vi "IMAQ-test.vi"() -> ()   [LabVIEW 2013]
uses:
  init & communication/Event.ctl
  init & communication/data-package.ctl
  init & communication/Event1.ctl
  init & communication/event-package.ctl
  init & communication/Setting.ctl
  init & communication/init-status.ctl
panel:
  in  "Status":T1 {"Setting"."X Pos." scale=-2.0..2.0; "Setting"."Y Pos." scale=-2.0..2.0}
  out "Image Out":T4(plugin-control)
  out "强度图":dbl[][](graph)
  in  "File Path":path
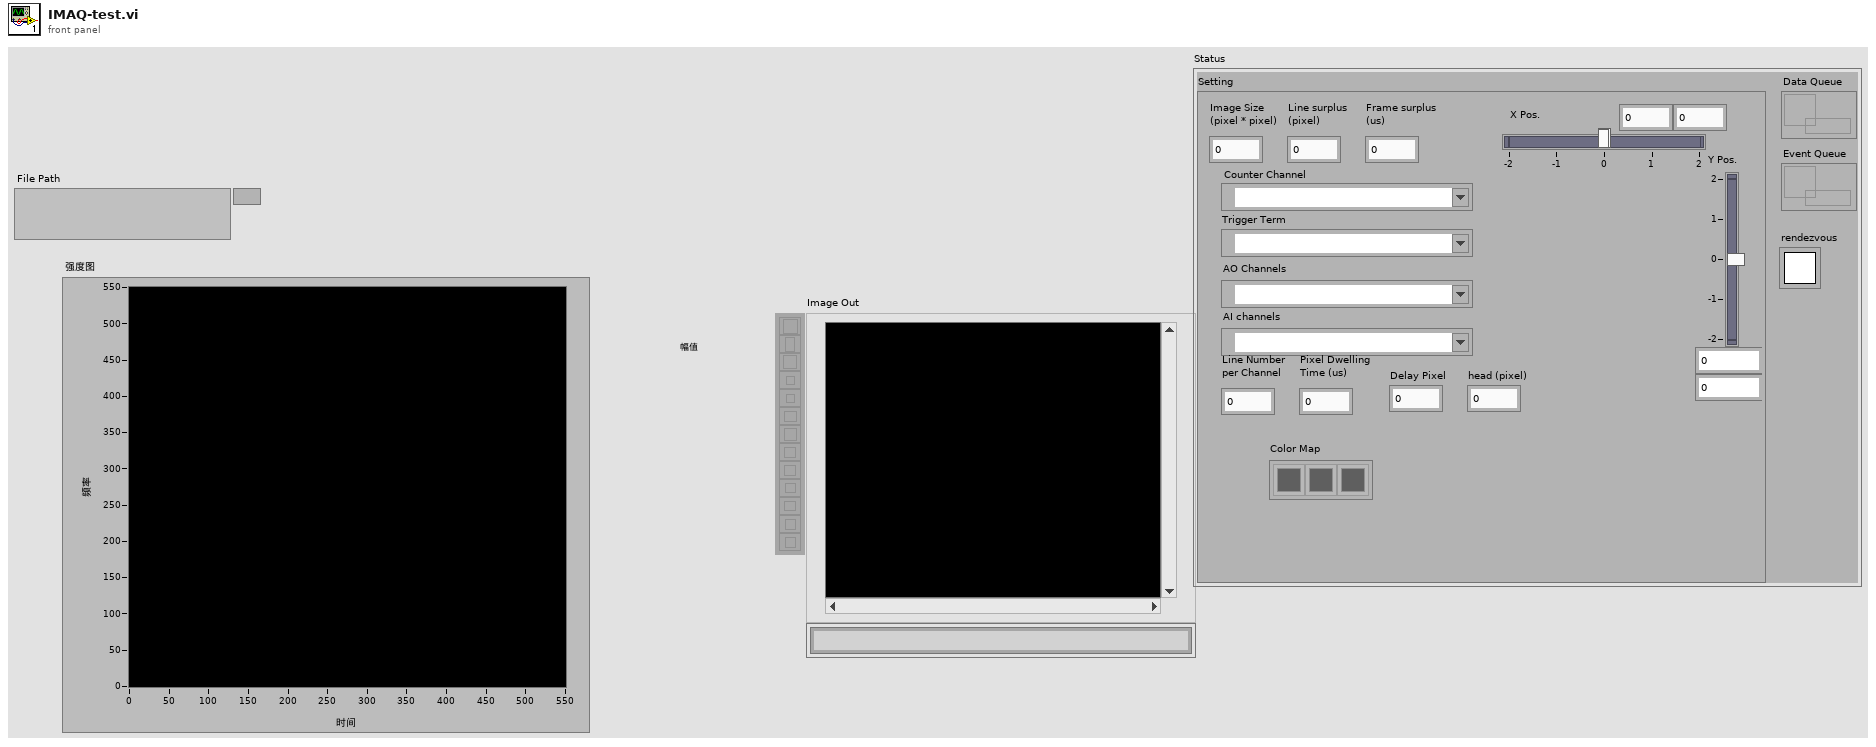
[diagram p1: front panel]
types:
  T1 = typedef "init-status.ctl" = cluster{"Setting":T2, "Event Queue":refnum<queue>, "Data Queue":refnum<queue>, "rendezvous":T3}
  T2 = typedef "Setting.ctl" = cluster{"Image Size\n(pixel * pixel)":i32, "Counter Channel":tag, "Trigger Term":tag, "AO Channels":tag, "Y Pos.":cluster{dbl, dbl}, "X Pos.":cluster{dbl, dbl}, "Line surplus\n(pixel)":i32, "Frame surplus\n(us)":i32, "AI channels":tag, "Line Number\nper Channel":i32, "Delay Pixel":i32, "Pixel Dwelling\nTime (us)":i32, "Color Map":u32[], "head (pixel)":i32}
  T3 = typedef "Rendezvous RefNum" = refnum<k1>
  T4 = typedef "IMAQ Image.ctl" = refnum<image>
  T5 = typedef "Image Type" = u32
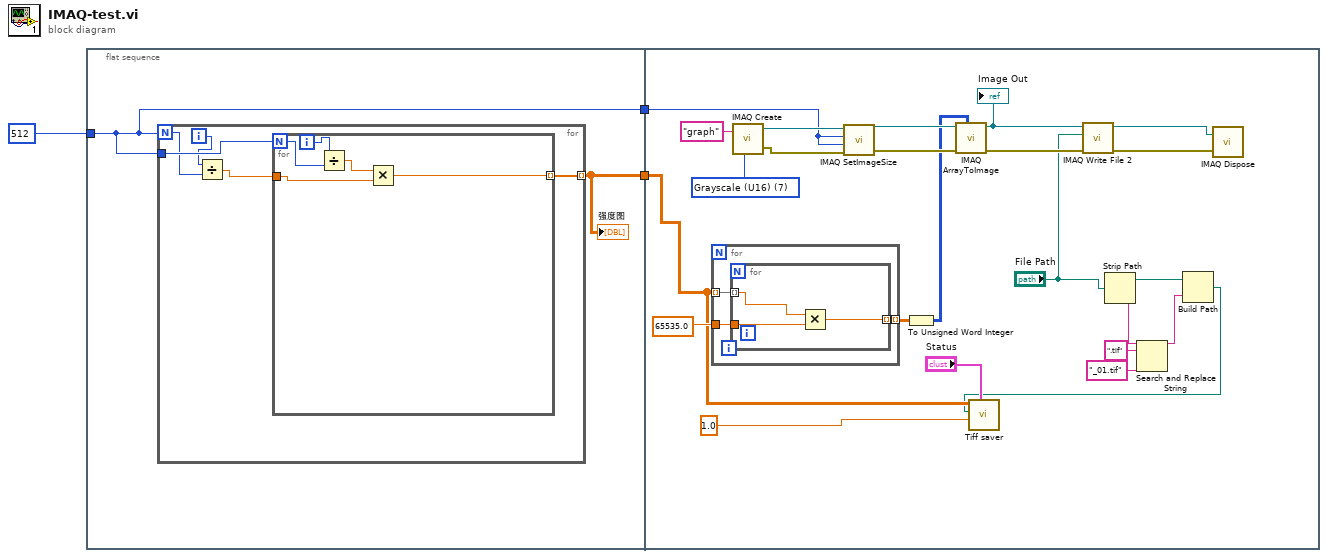
[diagram p0: block diagram]
diagram:
  n1 = flat-sequence {
    tunnel: 512 -> [w5]
    tunnel: [w4] -> w2
    tunnel: [w5] -> w1
    tunnel: w2 -> [w24]
    tunnel: w1 -> [w30]
    frame #0 {
      n2 = for {
        N: w5 -> [w9]
        tunnel: w5 -> [w10]
        tunnel: [w6] -> w4 mode=indexing
        i -> [w8]
        n3 = Divide(x=w8, y=w9) -> (x/y=w7:dbl)
        n4 = for {
          N: w10 -> [w11]
          tunnel: w7 -> [w14]
          tunnel: [w13] -> w6 mode=indexing
          i -> [w12]
          n5 = Divide(x=w12, y=w11) -> (x/y=w15:dbl)
          n6 = Multiply(x=w15, y=w14) -> (x*y=w13:dbl)
        }
      }
      "强度图" <- w4
    }
    frame #1 {
      w31 = T5 7 items=["Grayscale (U8)", "Grayscale (I16)", "Grayscale (SGL)", "Complex (CSG)", "RGB (U32)", "HSL (U32)", "RGB (U64)", "Grayscale (U16)"] ("Image Type")
      n7 = for {
        tunnel: w24 -> [w42] mode=indexing
        tunnel: 65535.0 -> [w41]
        tunnel: [w40] -> w27 mode=indexing
        n8 = for {
          tunnel: w42 -> [w45] mode=indexing
          tunnel: w41 -> [w44]
          tunnel: [w43] -> w40 mode=indexing
          n9 = Multiply(x=w45, y=w44) -> (x*y=w43:dbl)
        }
      }
      n10 = call "IMAQ Create"("Image Name"="graph", "Image Type"=w31) -> ("New Image"=w32:T4, "error out"=w38:errorcluster)  [unwired: 3 in]
      n11 = call "IMAQ SetImageSize"("error in (no error)"=w38, "Y Resolution"=w30, "X Resolution"=w30, "Image"=w32) -> ("error out"=w37:errorcluster, "Image Out"=w33:T4)  [unwired: 1 in]
      n12 = To Unsigned Word Integer(number=w27) -> (unsigned 16bit integer=w26:u16[][])
      n13 = call "IMAQ ArrayToImage"("Image Pixels (U16)"=w26, "error in (no error)"=w37, "Image"=w33) -> ("error out"=w36:errorcluster, "Image Out"=w29:T4)  [unwired: 7 in]
      "Image Out" <- w29
      n14 = call-poly "IMAQ Write File 2"("error in (no error)"=w36, "File Path"="File Path", "Image"=w29) -> ("error out"=w35:errorcluster, "Image Out (duplicate)"=w34:T4)  [unwired: 7 in]
      n15 = Strip Path(path="File Path") -> (stripped path=w21:path, name=w20:string)
      n16 = Search and Replace String(input string=w20, search string=".tif" ("搜索字符串"), replace string="_01.tif" ("替换字符串(\"\")")) -> (result string=w19:string)  [unwired: 5 in, 3 out]
      n17 = Build Path(base path=w21, name or relative path=w19) -> (appended path=w16:path)
      n18 = call "Tiff saver.vi"("Status"="Status", 9:1.0 ("Max Val"), "File Path"=w16, "Image in"=w24) -> ()  [unwired: 7 in, 1 out]
      n19 = call "IMAQ Dispose"("Image"=w34, "error in (no error)"=w35) -> ()  [unwired: 4 in, 1 out]
    }
  }
